vi "testcase - load and list configurations.vi"() -> ()   [LabVIEW 2017]
uses:
  INI-Static-Variable-Support/INI-Static-Variable-Support.lvlib
panel:
  out "all configurations 2":path[](array[path])
  out "Array 3":string[](array[string])
  out "Default Config File Path":path
  out "error out":errorcluster
  out "all configurations":path[](array[path])
  out "Array 2":string[](array[string])
  out "Array":cluster{"Value":string, "Array":string[]}[](array[cluster])
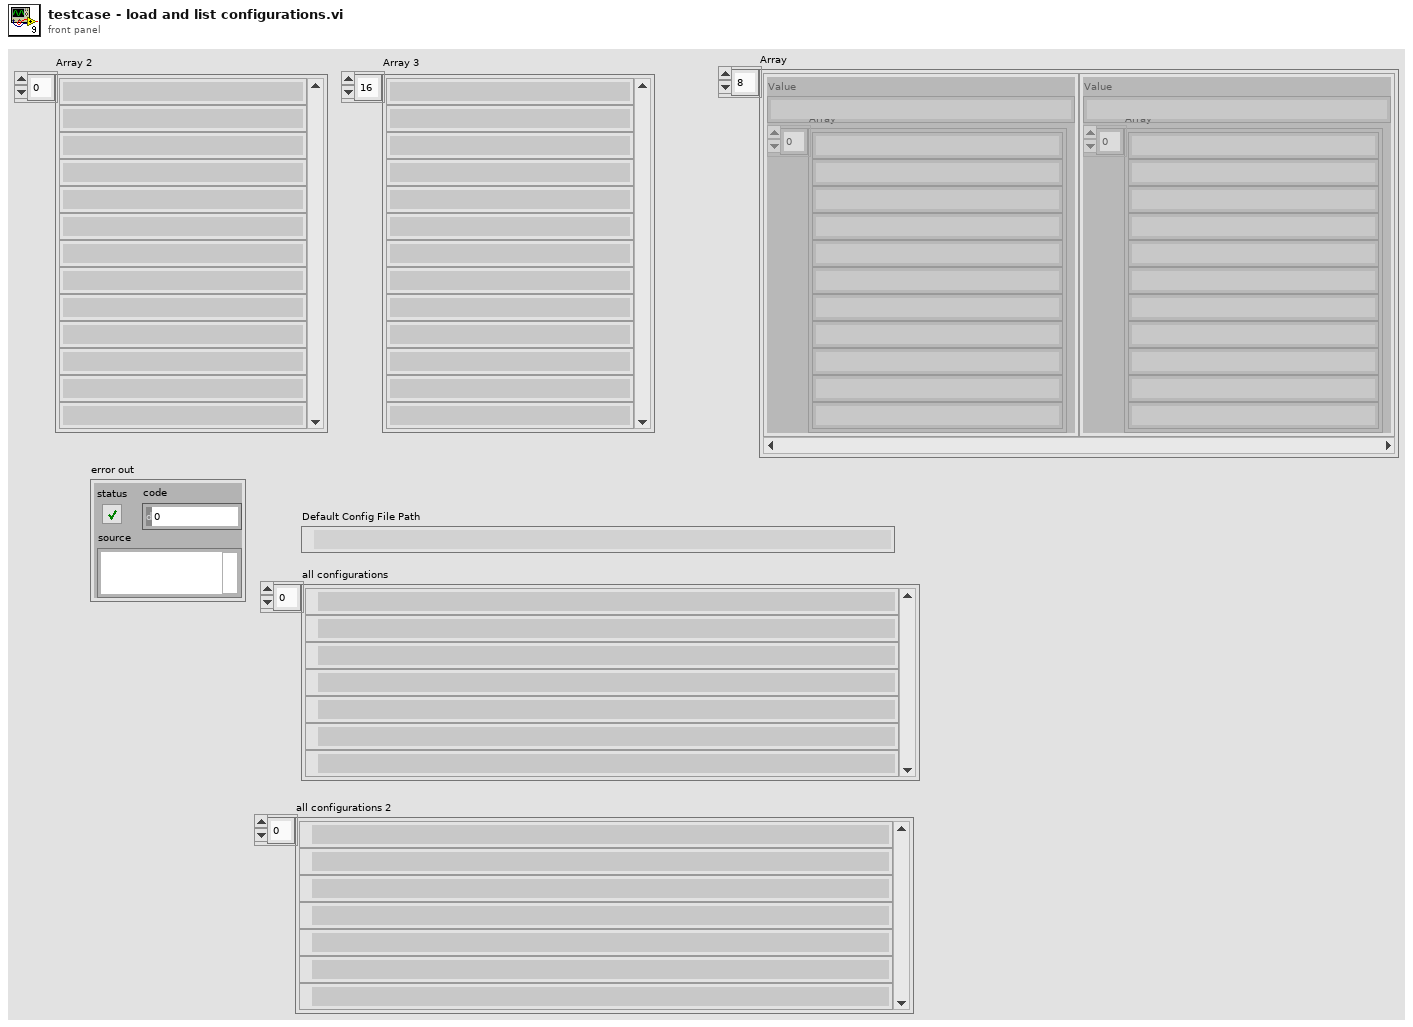
[diagram p1: front panel]
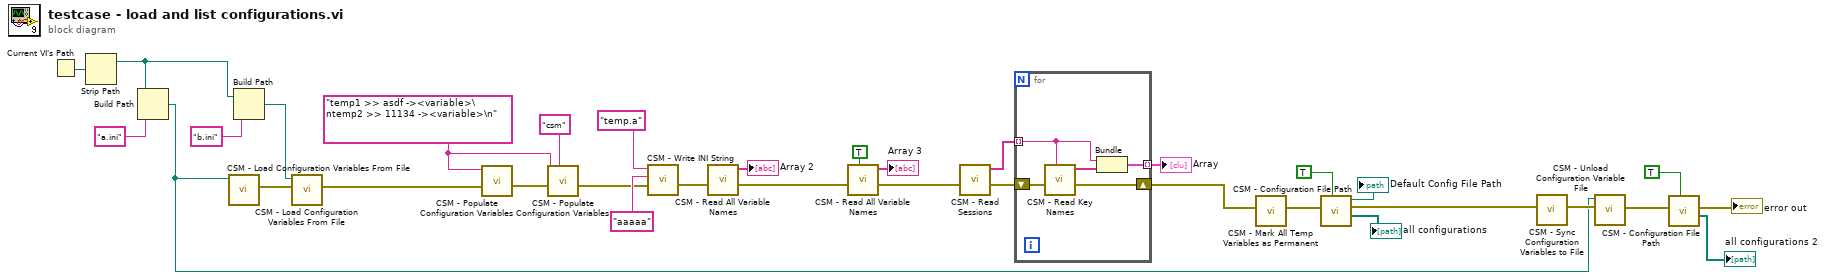
[diagram p0: block diagram]
diagram:
  w14 = "temp1 >> asdf -><variable>\ntemp2 >> 11134 -><variable>\n" ("String in")
  n1 = Current VI's Path() -> (path=w34:path)
  n2 = Strip Path(path=w34) -> (stripped path=w30:path)  [unwired: 1 out]
  n3 = Build Path(base path=w30, name or relative path="a.ini") -> (appended path=w5:path)
  n4 = call "CSM - Load Configuration Variables From File.vi"("Path"=w5) -> ("error out"=w32:errorcluster)  [unwired: 8 in]
  n5 = Build Path(base path=w30, name or relative path="b.ini") -> (appended path=w29:path)
  n6 = call "CSM - Load Configuration Variables From File.vi"("error in (no error)"=w32, "Path"=w29) -> ("error out"=w15:errorcluster)  [unwired: 7 in]
  n7 = call "CSM - Populate Configuration Variables.vi"("error in (no error)"=w15, "String in"=w14) -> ("error out"=w13:errorcluster)  [unwired: 6 in, 1 out]
  n8 = call "CSM - Populate Configuration Variables.vi"("Section Name(\"\" as Default)"="csm" ("Section Name(\"\" as Default)"), "error in (no error)"=w13, "String in"=w14) -> ("error out"=w12:errorcluster)  [unwired: 5 in, 1 out]
  n9 = call "CSM - Write INI String.vi"("error in (no error)"=w12, "String"="aaaaa" (">> Variable Name >>"), ">> Variable Name >>"="temp.a") -> ("error out"=w18:errorcluster)  [unwired: 5 in, 1 out]
  n10 = call "CSM - Read All Variable Names.vi"("error in (no error)"=w18) -> ("error out"=w21:errorcluster, "Array"=→"Array 2":string[])  [unwired: 7 in]
  n11 = call "CSM - Read All Variable Names.vi"("Permanent Variables Only?"=TRUE, "error in (no error)"=w21) -> ("error out"=w20:errorcluster, "Array"=→"Array 3":string[])  [unwired: 6 in]
  n12 = call "CSM - Read Sessions.vi"("error in (no error)"=w20) -> ("error out"=w28:errorcluster, "Array"=w27:string[])  [unwired: 6 in, 1 out]
  n13 = for {
    tunnel: w27 -> [w36] mode=indexing
    tunnel: [w37] -> w26 mode=indexing
    shift-right: [w35] -> w10
    shift-left: w28 -> [w39]
    n14 = call "CSM - Read Key Names.vi"("Section Name(\"\" as Default)"=w36, "error in (no error)"=w39) -> ("error out"=w35:errorcluster, "Array"=w38:string[])  [unwired: 5 in, 1 out]
    n15 = Bundle("Value"=w36, "Array"=w38) -> (w37:cluster{"Value":string, "Array":string[]})  [unwired: 1 in]
  }
  "Array" <- w26
  n16 = call "CSM - Mark All Temp Variables as Permanent.vi"("error in (no error)"=w10) -> ("error out"=w9:errorcluster)  [unwired: 8 in]
  n17 = call "CSM - Configuration File Path.vi"("Include All Paths?(F)"=TRUE, "error in (no error)"=w9) -> ("All Config Files"=→"all configurations":path[], "error out"=w8:errorcluster, "Default Config File Path"=→"Default Config File Path":path)  [unwired: 5 in]
  n18 = call "CSM - Sync Configuration Variables to File.vi"("error in (no error)"=w8) -> ("error out"=w7:errorcluster)  [unwired: 8 in]
  n19 = call "CSM - Unload Configuration Variable File.vi"("error in (no error)"=w7, "Path"=w5) -> ("error out"=w3:errorcluster)  [unwired: 7 in]
  n20 = call "CSM - Configuration File Path.vi"("Include All Paths?(F)"=TRUE, "error in (no error)"=w3) -> ("All Config Files"=→"all configurations 2":path[], "error out"=→"error out":errorcluster)  [unwired: 5 in, 1 out]
